vi "Self-Test.vi"(8 "error in (no error)":errorcluster, 11 "VISA resource name":refnum<visa-resource-name>) -> (0 "error out":errorcluster, 1 "Vin reading":string, 2 "Self-Test Result Code":dbl, 3 "VISA resource name out":refnum<visa-resource-name>)   [LabVIEW 2012]
doc: "Runs the instrument's self-test routine and returns the test results."
panel:
  out "read buffer":string
  out "Pin reading":string
  out "Output pressure":dbl
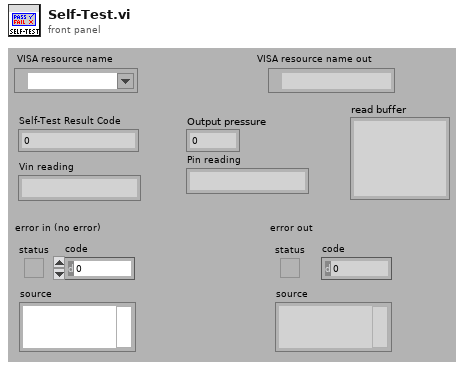
[diagram p1: front panel]
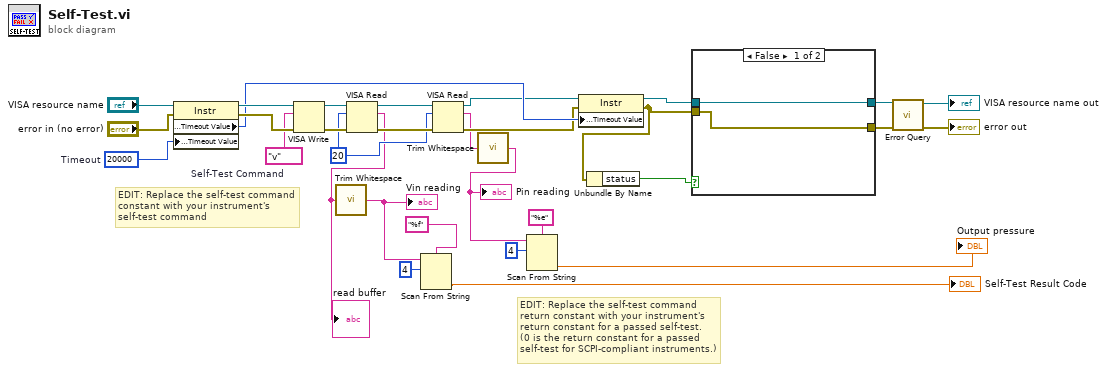
[diagram p0: block diagram]
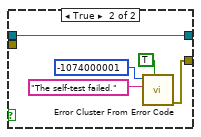
[diagram p2: hidden frame]
diagram:
  w12 = u32 20 ("byte count (20)")
  w25 = u32 20000  # Timeout
  w21 = "v"  # Self-Test Command
  # "EDIT: Replace the self-test command\nreturn constant with your instrument's \nreturn constant for a passed self-test.\n(0 is the return constant for a passed \nself-test for SCPI-compliant instruments.)"
  # "EDIT: Replace the self-test command\nconstant with your instrument's\nself-test command"
  n1 = property class="Instr"(reference="VISA resource name", error in="error in (no error)", "General Settings:Timeout Value"=w25) -> (reference out=w23:refnum<visa-resource-name>, error out=w24:errorcluster, "General Settings:Timeout Value"=w22:u32)
  n2 = VISA Write(VISA resource name=w23, write buffer=w21, error in (no error)=w24) -> (VISA resource name out=w31:refnum<visa-resource-name>, error out=w30:errorcluster)  [unwired: 1 out]
  n3 = VISA Read(VISA resource name=w31, byte count=w12, error in (no error)=w30) -> (VISA resource name out=w13:refnum<visa-resource-name>, read buffer=w4:string, error out=w16:errorcluster)  [unwired: 1 out]
  "read buffer" <- w4
  n4 = call <vilib>:"Trim Whitespace.vi"("string"=w4) -> ("trimmed string"=w3:string)  [unwired: 1 in]
  "Vin reading" <- w3
  n5 = Scan From String(format string="%f", input string=w3, initial scan location=u32 4) -> (output 1=→"Self-Test Result Code":dbl)  [unwired: 2 in, 3 out]
  n6 = VISA Read(VISA resource name=w13, byte count=w12, error in (no error)=w16) -> (VISA resource name out=w14:refnum<visa-resource-name>, read buffer=w2:string, error out=w15:errorcluster)  [unwired: 1 out]
  n7 = call <vilib>:"Trim Whitespace.vi"("string"=w2) -> ("trimmed string"=w1:string)  [unwired: 1 in]
  "Pin reading" <- w1
  n8 = Scan From String(format string="%e", input string=w1, initial scan location=u32 4) -> (output 1=→"Output pressure":dbl)  [unwired: 2 in, 3 out]
  n9 = property class="Instr"(reference=w14, error in=w15, "General Settings:Timeout Value"=w22) -> (reference out=w20:refnum<visa-resource-name>, error out=w19:errorcluster)
  n10 = Unbundle By Name(w19) -> ("status"=w9:bool)
  n11 = case shown="False" w9 {
    tunnel: w20 -> [w33 w38]
    tunnel: w19 -> [w32 _]
    tunnel: [w32 w34] -> w18
    tunnel: [w33 w38] -> w17
    frame False {
    }
    frame True {
      n12 = call <vilib>:"Error Cluster From Error Code.vi"("show call chain? (False)"=TRUE, "error message (\"\")"="The self-test failed." ("Source (VI Name)"), "error code (0)"=-1074000001 ("Code")) -> ("error out"=w34:errorcluster)  [unwired: 6 in]
    }
  }
  n13 = call <instrlib>:"Error Query.vi"("error in (no error)"=w18, "VISA resource name"=w17) -> ("error out"=→"error out":errorcluster, "VISA resource name out"=→"VISA resource name out":refnum<visa-resource-name>)  [unwired: 8 in]
